vi "Remove.vi"(8 "error in (no error)":errorcluster, 10 "Key":string, 11 "VariantAttribute in":refnum<class "MapImp.lvclass">) -> (0 "error out":errorcluster, 1 "Value":refnum<class>, 3 "VariantAttribute out":refnum<class "MapImp.lvclass">)   [LabVIEW 2013, in "LapDog.Collections.v1.Maps.lvlib" / "MapImp.lvclass"]
doc: "Removes the key-value pair from the collection.\n\nIf the key does not exist, error 510203 is returned."
uses:
  MapImp.lvclass
  MapImp.lvclass/MapImp.ctl
  LapDog.Collections.Common/LapDog.Collections.v1.Common.lvlib
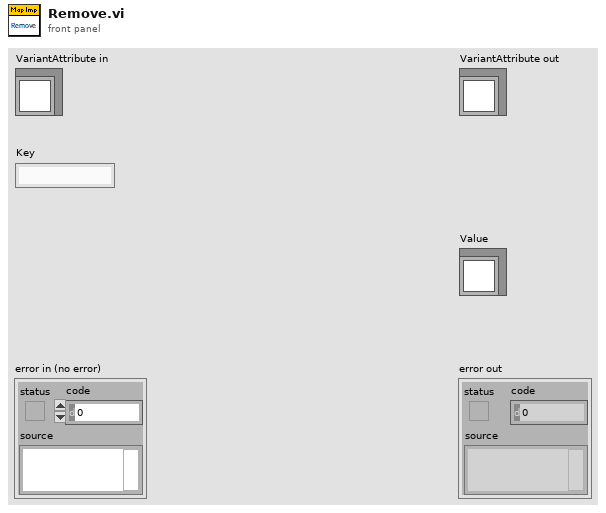
[diagram p1: front panel]
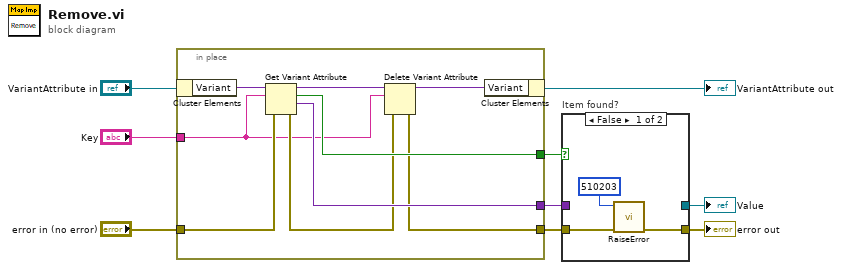
[diagram p0: block diagram]
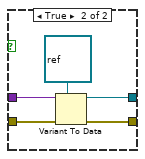
[diagram p2: hidden frame]
diagram:
  n1 = in-place {
    in-place-border: "error in (no error)" -> [w17]
    in-place-border: [w11] -> w4
    in-place-border: "Key" -> [w10]
    in-place-border: [w16] -> w1
    in-place-border: [w15] -> w3
    n2 = in-place-cluster #1("VariantAttribute in") -> ("Variant"=w18:variant)
    n3 = Get Variant Attribute(Variant=w18, name=w10, error in=w17) -> (duplicate Variant=w14:variant, found=w16:bool, value=w15:variant, error out=w12:errorcluster)  [unwired: 1 in]
    n4 = Delete Variant Attribute(4:w12, 6:w10, 7:w14) -> (0:w11:errorcluster, 3:w13:variant)  [unwired: 1 out]
    n5 = in-place-cluster #1("Variant"=w13) -> (→"VariantAttribute out":refnum<class "MapImp.lvclass">)
  }
  n6 = case "Item found?" shown="False" w1 {
    tunnel: [w20 w26] -> w5
    tunnel: w4 -> [w21 w25]
    tunnel: w3 -> [_ w24]
    tunnel: [_ w23] -> w2
    frame False {
      n7 = call "RaiseError.vi"("error in (no error)"=w21, "Error Code"=510203) -> ("error out"=w20:errorcluster)  [unwired: 9 in]
    }
    frame True {
      n8 = Variant To Data(error in=w25, type=refnum<class> refnum, Variant=w24) -> (data=w23:refnum<class>, error out=w26:errorcluster)
    }
  }
  "error out" <- w5
  "Value" <- w2
